vi "Reinit All Element Values.vi"(8 "error in":errorcluster, 11 "Class in":refnum<class>) -> (0 "error out":errorcluster, 3 "Class out":refnum<class>)   [LabVIEW 2023, in "Label-Driven UI.lvlib"]
doc: "VI가 가진 모든 값을 기본값으로 초기화합니다."
uses:
  Label-Driven UI.lvlib
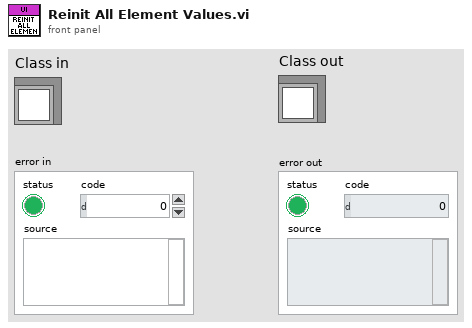
[diagram p1: front panel]
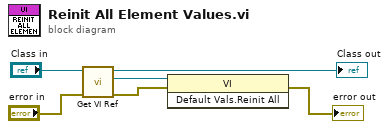
[diagram p0: block diagram]
diagram:
  n1 = call "Get VI Ref.vi"("error in"="error in", "Class in"="Class in") -> ("error out"=w4:errorcluster, "VI Refnum"=w5:refnum<vi>, "Class out"=→"Class out":refnum<class>)  [unwired: 7 in]
  n2 = invoke class="VI" method="Default Vals.Reinit All"(reference=w5, error in=w4) -> (error out=→"error out":errorcluster)  [unwired: 1 in, 2 out]
